vi "曲线模型计算.vi"(11 "曲线模型":T2={"标液浓度1"=0.0, "测量吸光度1"=0.0, "样品1启用"=FALSE, "标液浓度2"=0.0, "测量吸光度2"=0.0, "样品2启用"=FALSE, "标液浓度3"=0.0, "测量吸光度3"=0.0, "样品3启用"=FALSE, "标液浓度4"=0.0, "测量吸光度4"=0.0, "样品4启用"=FALSE, "标液浓度5"=0.0, "测量吸光度5"=0.0, "样品5启用"=FALSE, "模型"=enum."线性", "精度"=4.0, "XY图"=[], "拟合公式"="", "r^2"=0.0, "标样一校准时间"=timestamp(0 s since 1904-01-01), "标样二校准时间"=timestamp(0 s since 1904-01-01), "标样三校准时间"=timestamp(0 s since 1904-01-01), "标样四校准时间"=timestamp(0 s since 1904-01-01), "标样五校准时间"=timestamp(0 s since 1904-01-01), "二次方程"={"x^2"=0.0, "K"=0.0, "B"=0.0}, "标定时间"=timestamp(0 s since 1904-01-01), "拟合公式 2"="", "r^2 2"=0.0} {"r^2 2" format="%.7f"; "标定时间" format="%<%Y/%m/%d %H:%M:%S>T"; "标样五校准时间" format="%<%Y/%m/%d %H:%M:%S>T"; "标样四校准时间" format="%<%Y/%m/%d %H:%M:%S>T"; "标样三校准时间" format="%<%Y/%m/%d %H:%M:%S>T"; "标样二校准时间" format="%<%Y/%m/%d %H:%M:%S>T"; "标样一校准时间" format="%<%Y/%m/%d %H:%M:%S>T"; "r^2" format="%.7f"; "测量吸光度5" format="%#.6f"; "测量吸光度4" format="%#.6f"; "测量吸光度3" format="%#.6f"; "测量吸光度2" format="%#.6f"; "测量吸光度1" format="%#.6f"}) -> (1 "公式切换阈值滴定数(0~9999)":dbl, 2 "二次方程 2":cluster{"x^2":dbl, "K":dbl, "B":dbl}, 3 "输出簇":T1)   [LabVIEW 2016, in "斯坦道CODMn新电路板.lvlib"]
uses:
  <vilib>/Analysis/6fits.llb/Curve Fitting Criteria.ctl
  <vilib>/Analysis/NI_AALPro.lvlib
panel:
  # "校准时间"
  # "标液浓度"
  # "滴定数"
  # "标液一"
  # "标液二"
  # "标液三"
  # "零点"
  # "跨度"
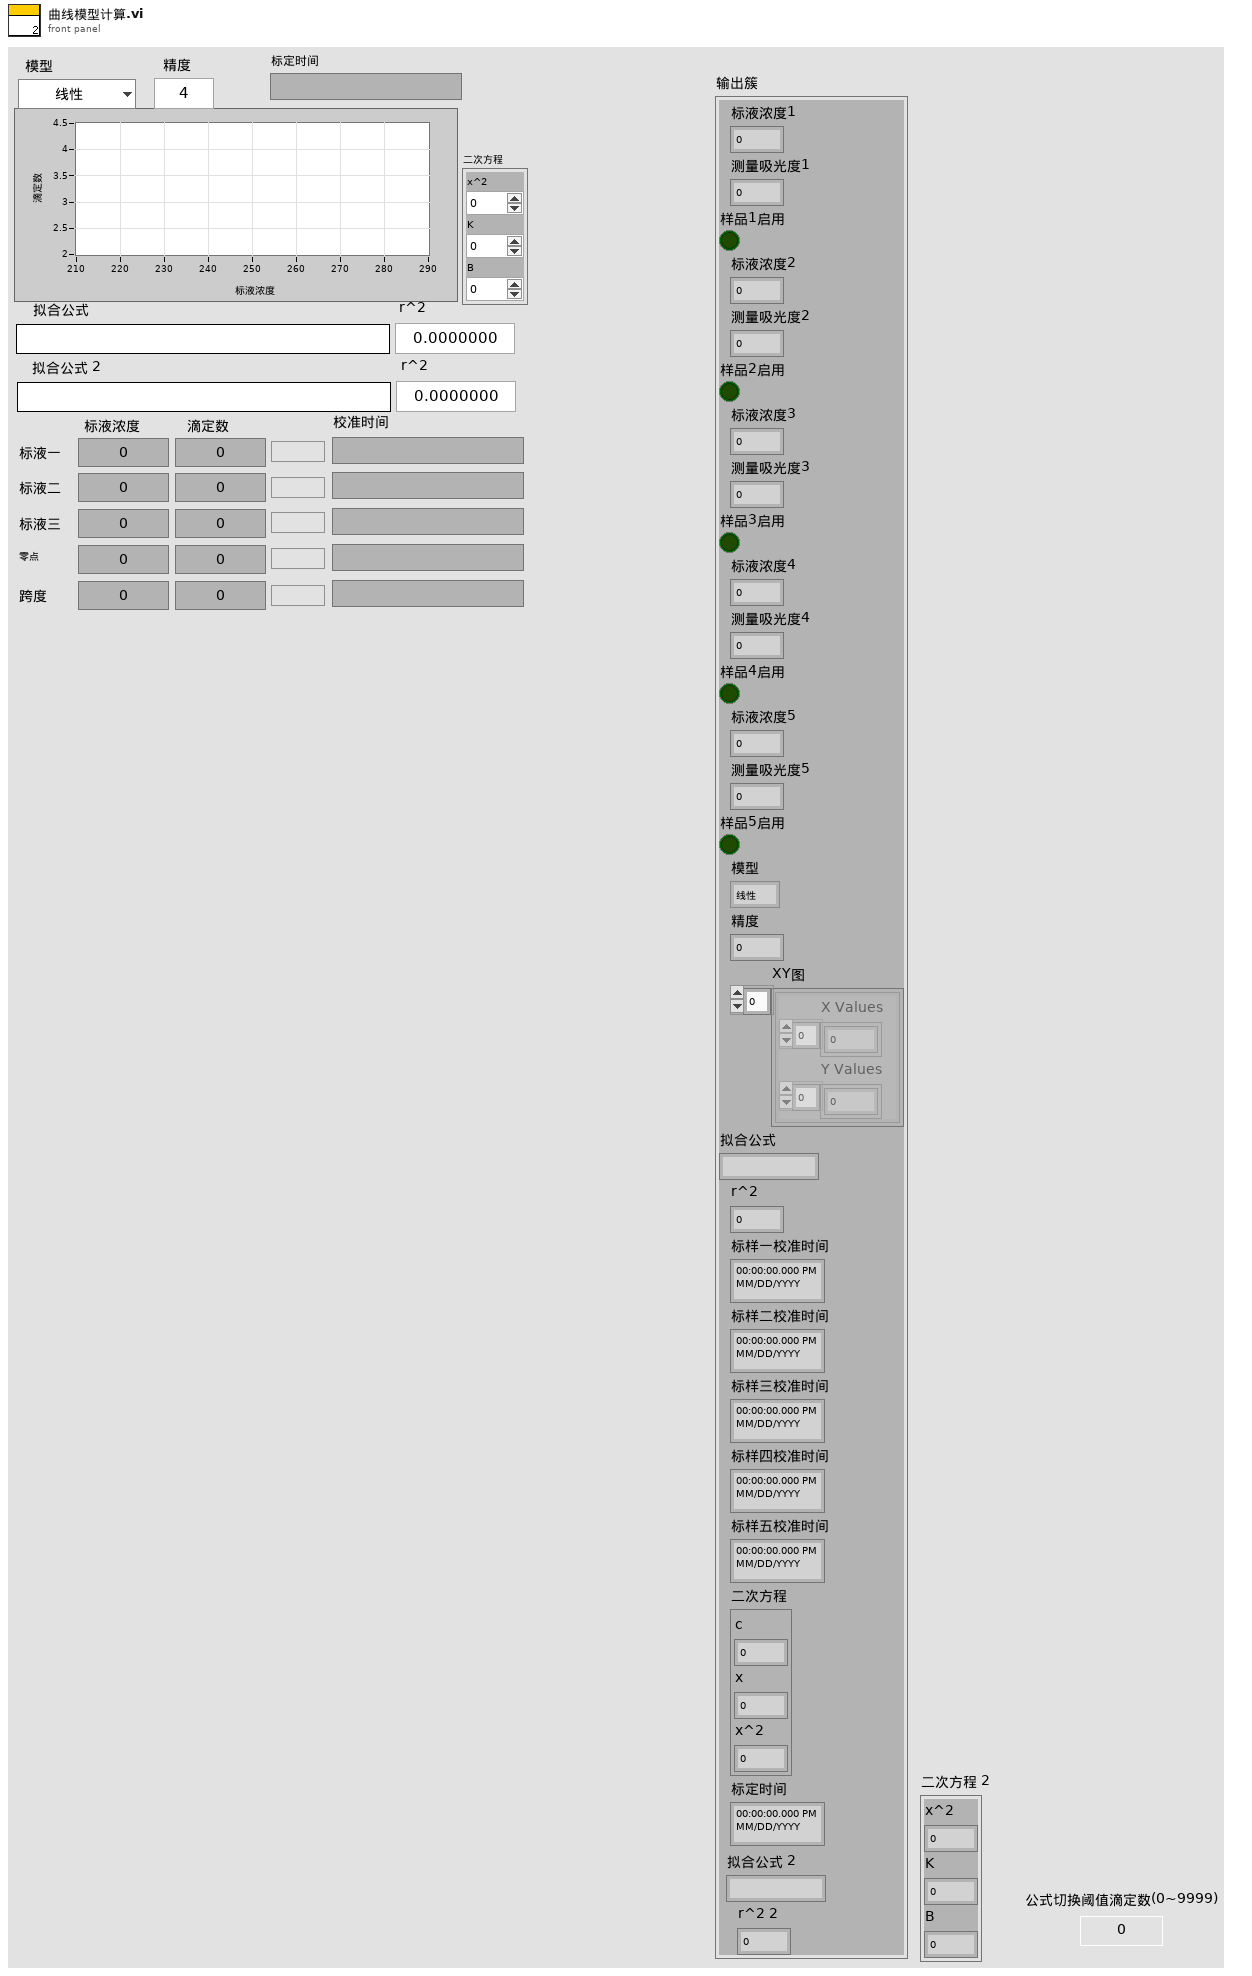
[diagram p1: front panel]
types:
  T1 = cluster{"标液浓度1":dbl, "测量吸光度1":dbl, "样品1启用":bool, "标液浓度2":dbl, "测量吸光度2":dbl, "样品2启用":bool, "标液浓度3":dbl, "测量吸光度3":dbl, "样品3启用":bool, "标液浓度4":dbl, "测量吸光度4":dbl, "样品4启用":bool, "标液浓度5":dbl, "测量吸光度5":dbl, "样品5启用":bool, "模型":enum32{"线性", "多项式", "折线"}, "精度":dbl, "XY图":cluster{"X Values":dbl[], "Y Values":dbl[]}[], "拟合公式":string, "r^2":dbl, "标样一校准时间":timestamp, "标样二校准时间":timestamp, "标样三校准时间":timestamp, "标样四校准时间":timestamp, "标样五校准时间":timestamp, "二次方程":cluster{"c":dbl, "x":dbl, "x^2":dbl}, "标定时间":timestamp, "拟合公式 2":string, "r^2 2":dbl}
  T2 = cluster{"标液浓度1":dbl, "测量吸光度1":dbl, "样品1启用":bool, "标液浓度2":dbl, "测量吸光度2":dbl, "样品2启用":bool, "标液浓度3":dbl, "测量吸光度3":dbl, "样品3启用":bool, "标液浓度4":dbl, "测量吸光度4":dbl, "样品4启用":bool, "标液浓度5":dbl, "测量吸光度5":dbl, "样品5启用":bool, "模型":enum32{"线性", "多项式", "折线"}, "精度":dbl, "XY图":cluster{"X Values":dbl[], "Y Values":dbl[]}[], "拟合公式":string, "r^2":dbl, "标样一校准时间":timestamp, "标样二校准时间":timestamp, "标样三校准时间":timestamp, "标样四校准时间":timestamp, "标样五校准时间":timestamp, "二次方程":cluster{"x^2":dbl, "K":dbl, "B":dbl}, "标定时间":timestamp, "拟合公式 2":string, "r^2 2":dbl}
  T3 = typedef "NI_AALPro.lvlib/Curve Fitting Criteria.ctl" = u16
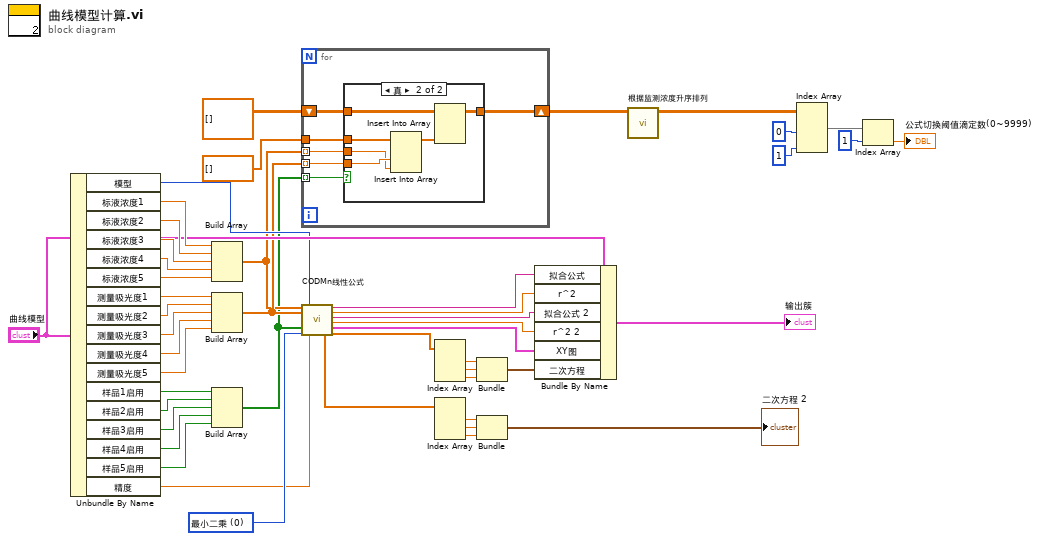
[diagram p0: block diagram]
diagram:
  w32 = T3 0 items=["最小二乘", "最小绝对残差", "Bisquare"] ("method")
  n1 = Unbundle By Name("曲线模型") -> ("模型"=w13:enum32{"线性", "多项式", "折线"}, "标液浓度1"=w47:dbl, "标液浓度2"=w46:dbl, "标液浓度3"=w45:dbl, "标液浓度4"=w44:dbl, "标液浓度5"=w43:dbl, "测量吸光度1"=w42:dbl, "测量吸光度2"=w41:dbl, "测量吸光度3"=w40:dbl, "测量吸光度4"=w39:dbl, "测量吸光度5"=w38:dbl, "样品1启用"=w37:bool, "样品2启用"=w36:bool, "样品3启用"=w35:bool, "样品4启用"=w34:bool, "样品5启用"=w33:bool, "精度"=w31:dbl)
  n2 = Build Array(w47, w46, w45, w44, w43) -> (w8:dbl[])
  n3 = Build Array(w42, w41, w40, w39, w38) -> (w9:dbl[])
  n4 = Build Array(w37, w36, w35, w34, w33) -> (w7:bool[])
  n5 = for {
    tunnel: w7 -> [w48] mode=indexing
    tunnel: w9 -> [w51] mode=indexing
    tunnel: w8 -> [w50] mode=indexing
    shift-right: [w49] -> w10
    shift-left: dbl[][] [] ("标液浓度") -> [w53]
    tunnel: dbl[] [] ("监测浓度") -> [w52]
    n6 = case shown="真" w48 {
      tunnel: w53 -> [w54 w60]
      tunnel: w52 -> [_ w59]
      tunnel: w51 -> [_ w58]
      tunnel: w50 -> [_ w57]
      tunnel: [w54 w55] -> w49
      frame False {
      }
      frame True {
        n7 = Insert Into Array(array=w59, new element #1=w58, new element #2=w57) -> (w56:dbl[])  [unwired: 1 in]
        n8 = Insert Into Array(array=w60, new element=w56) -> (w55:dbl[][])  [unwired: 2 in]
      }
    }
  }
  n9 = call "CODMn线性公式.vi"("标液浓度"=w8, "信号值"=w9, "启用"=w7, "method"=w32, "模型"=w13, "精度"=w31) -> ("Polynomial Coefficients 2"=w17:dbl[], "拟合方程"=w30:string, "r^2"=w29:dbl, "拟合方程 2"=w28:string, "r^2 2"=w27:dbl, "XY图"=w26:cluster{"X Values":dbl[], "Y Values":dbl[]}[], "Polynomial Coefficients"=w22:dbl[])  [unwired: 7 in]
  n10 = Index Array(array=w22) -> (element #1=w25:dbl, element #2=w24:dbl, element #3=w23:dbl)  [unwired: 3 in]
  n11 = Index Array(array=w17) -> (element #1=w18:dbl, element #2=w19:dbl, element #3=w20:dbl)  [unwired: 3 in]
  n12 = Bundle("数值"=w25, "数值"=w24, "数值"=w23) -> (w21:cluster{"数值":dbl, "数值":dbl, "数值":dbl})  [unwired: 1 in]
  n13 = Bundle("数值"=w18, "数值"=w19, "数值"=w20) -> (→"二次方程 2":cluster{"数值":dbl, "数值":dbl, "数值":dbl})  [unwired: 1 in]
  n14 = Bundle By Name(cluster="曲线模型", "拟合公式"=w30, "r^2"=w29, "拟合公式 2"=w28, "r^2 2"=w27, "XY图"=w26, "二次方程"=w21) -> (→"输出簇":T2)
  n15 = call "根据监测浓度升序排列.vi"("标液浓度输入"=w10) -> ("输出数组"=w4:dbl[][])  [unwired: 10 in]
  n16 = Index Array(array=w4, index (col) #1=0 ("禁用的索引 (列)"), index (col) #2=1 ("索引 (列)")) -> (element #1=w2:dbl[])  [unwired: 2 in, 1 out]
  n17 = Index Array(array=w2, index=1 ("索引")) -> (element=→"公式切换阈值滴定数(0~9999)":dbl)
